vi "Scan action.vi"(8 "error in (no error)":errorcluster, 11 "SweepControl in":refnum<class "SMO.SweepControl.lvclass">) -> (0 "error out":errorcluster, 1 "Stop?":bool, 3 "SweepControl out":refnum<class "SMO.SweepControl.lvclass">)   [LabVIEW 2019, in "SMO.SweepControl.lvclass"]
uses:
  SMO.SweepControl.lvclass
  <userlib>/LevyLab/Lockin-Multichannel/Instrument.Lockin/Instrument.Lockin.lvclass
  Control Experiment/Control Experiment.lvclass
  <userlib>/LevyLab/Instrument Framework/Instrument Types/Cryostat/Typedefs/Magnet Mode--Enum.ctl
  <userlib>/LevyLab/Instrument Framework/Instrument Types/Cryostat/Instrument.Cryostat.lvclass
  <userlib>/LevyLab/Instrument Framework/Instrument Types/Strain/Instrument.Strain.lvclass
  <userlib>/LevyLab/Instrument Framework/Instrument Types/Delay Line/Instrument.DelayLine.lvclass
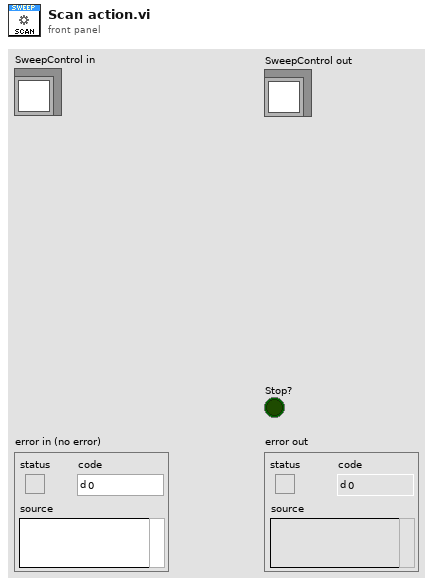
[diagram p1: front panel]
types:
  T1 = typedef "SMO.SweepControl.lvclass/Cluster - Sweep Control.ctl" = cluster{"Start":dbl, "End":dbl, "Step":dbl, "Rate":dbl, "wait (ms/mK)":u32, "Address":string, "Priority":T2, "Scan name":T3, "Post Actions":T4[], "channel":i32}
  T2 = typedef "SMO.SweepControl.lvclass/Enum - Priority.ctl" = enum16{"Priority 0", "Priority 1", "Priority 2", "Priority 3", "Priority 4", "Priority 5"}
  T3 = typedef "SMO.SweepControl.lvclass/Enum - Action.ctl" = enum16{"OFF", "time", "Lockin Amplitude", "Lockin Frequency", "Lockin Bias", "Delay", "Strain", "DAQ Bias", "Magnet Field", "Temperature", "MW f1", "MW f2", "MW Amplitude1", "MW Amplitude2"}
  T4 = typedef "SMO.SweepControl.lvclass/Enum - PostAction - 2.ctl" = enum16{"Do Nothing", "Wait (time)", "Wait (Temperature)", "Wait (<T ; B sweep)", "Wait (Magnet)"}
  T5 = typedef "SMO.SweepControl.lvclass/ScanParamters.ctl" = T6[]
  T6 = typedef "SMO.SweepControl.lvclass/Cluster - ScanParamters.ctl" = cluster{"Start":dbl, "End":dbl, "Step":dbl, "Rate":dbl, "Waveform type":enum16{"linear", "triangle", "power"}, "wait (ms or K)":dbl, "Address":string, "channel":i32}
  T7 = typedef "SMO.SweepControl.lvclass/ScanControl.ctl" = T8[]
  T8 = typedef "SMO.SweepControl.lvclass/Cluster - ScanControl.ctl" = cluster{"Priority":T2, "Scan name":T3}
  T9 = typedef "Control Experiment.lvclass/Instruments--cluster.ctl" = cluster{"KH7008":refnum<class "Instrument.KH7008.lvclass">[], "Lockin":refnum<class "Instrument.Lockin.lvclass">, "Temperature":refnum<class "Instrument.Cryostat.lvclass">, "Magnet":refnum<class "Instrument.Cryostat.lvclass">, "Rotator":refnum<class "Instrument.Cryostat.lvclass">, "Level":refnum<class "Instrument.Cryostat.lvclass">, "Capacitance Bridge":refnum<class "Instrument.CBridge.lvclass">, "Delay Line":refnum<class "Instrument.DelayLine.lvclass">, "Strain Cell":refnum<class "Instrument.Strain.lvclass">, "VNA":refnum<class "Instrument.VNA.lvclass">, "Voltage Source":refnum<class "Instrument.VSource.lvclass">}
  T10 = typedef "Instrument.Cryostat.lvclass/Magnet Mode--Enum.ctl" = enum16{"Persistent", "Driven"}
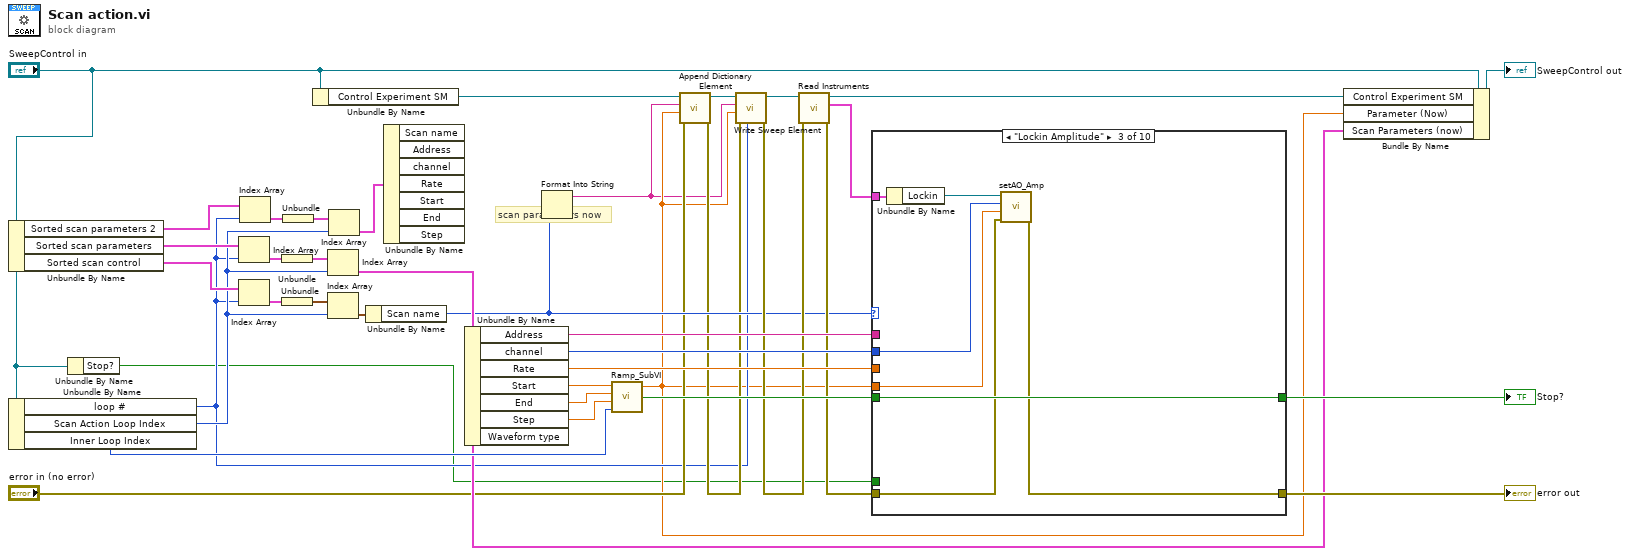
[diagram p0: block diagram]
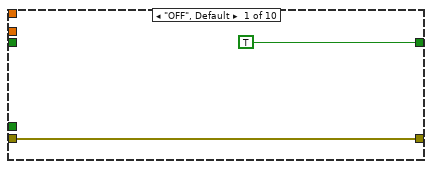
[diagram p2: hidden frame]
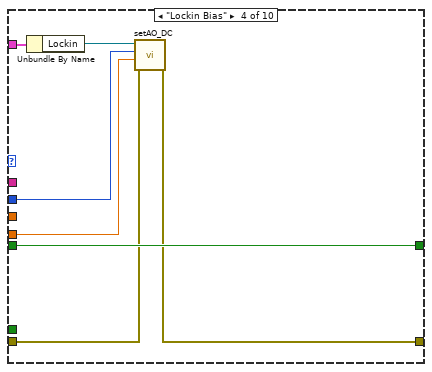
[diagram p4: hidden frame]
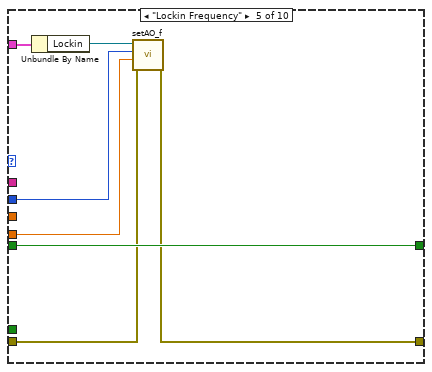
[diagram p5: hidden frame]
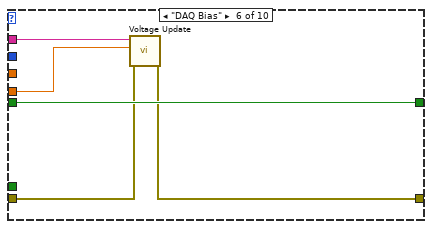
[diagram p6: hidden frame]
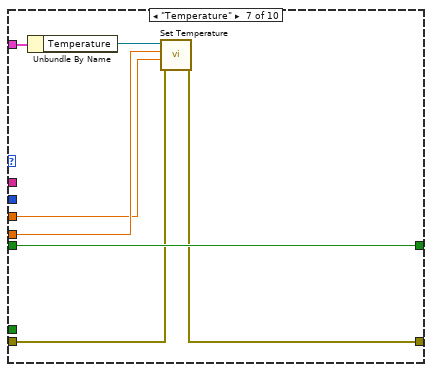
[diagram p7: hidden frame]
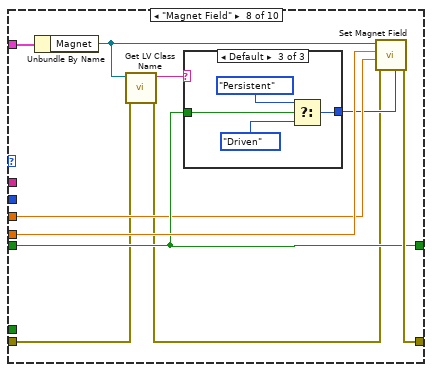
[diagram p8: hidden frame]
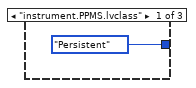
[diagram p9: hidden frame]
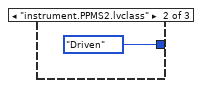
[diagram p10: hidden frame]
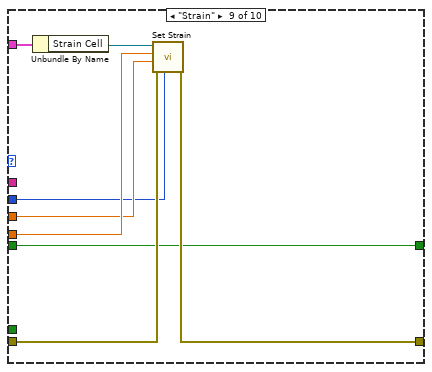
[diagram p11: hidden frame]
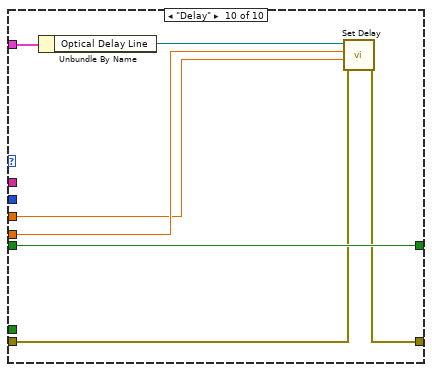
[diagram p12: hidden frame]
diagram:
  # "scan parameters now"
  n1 = Unbundle By Name("SweepControl in") -> ("Sorted scan parameters 2"=w13:cluster{"Scan parameters 2":T1[]}[], "Sorted scan parameters"=w30:cluster{T5}[], "Sorted scan control"=w24:cluster{T7}[])
  n2 = Unbundle By Name("SweepControl in") -> ("loop #"=w6:i32, "Scan Action Loop Index"=w14:i32, "Inner Loop Index"=w31:i32)
  n3 = Unbundle By Name("SweepControl in") -> ("Stop?"=w1:bool)
  n4 = Index Array(array=w30, index=w6) -> (element=w29:cluster{T5})
  n5 = Index Array(array=w24, index=w6) -> (element=w26:cluster{T7})
  n6 = Index Array(array=w13, index=w6) -> (element=w15:cluster{"Scan parameters 2":T1[]})
  n7 = Unbundle(w29) -> (w28:T5)
  n8 = Unbundle(w26) -> (w27:T7)
  n9 = Unbundle(w15) -> ("Scan parameters 2"=w16:T1[])
  n10 = Unbundle By Name("SweepControl in") -> ("Control Experiment SM"=w9:refnum<class "Control Experiment SM.lvclass">)
  n11 = Index Array(array=w28, index=w14) -> (element=w11:T6)
  n12 = Index Array(array=w27, index=w14) -> (element=w25:T8)
  n13 = Index Array(array=w16, index=w14) -> (element=w12:T1)
  n14 = Unbundle By Name(w25) -> ("Scan name"=w10:T3)
  n15 = Unbundle By Name(w12) -> ()  [unwired: 7 out]
  n16 = Unbundle By Name(w11) -> ("Address"=w37:string, "channel"=w39:i32, "Rate"=w34:dbl, "Start"=w36:dbl, "End"=w23:dbl, "Step"=w22:dbl)  [unwired: 1 out]
  n17 = Format Into String(w10) -> (resulting string=w3:string)  [unwired: 3 in, 1 out]
  n18 = call <userlib>:"Ramp_SubVI.vi"("index"=w31, "step"=w22, "end"=w23, "start"=w36) -> ("Stop?"=w35:bool, "Numeric"=w4:dbl)  [unwired: 1 in]
  n19 = call "Append Dictionary Element.vi"("error in (no error)"="error in (no error)", "value"=w4, "key"=w3, "Control Experiment in"=w9) -> ("error out"=w7:errorcluster, "Control Experiment out"=w5:refnum<class "Control Experiment.lvclass">)  [unwired: 6 in]
  n20 = call "Write Sweep Element.vi"("loop index"=w6, "error in (no error)"=w7, "value"=w4, "key"=w3, "Control Experiment in"=w5) -> ("error out"=w20:errorcluster, "Control Experiment out"=w21:refnum<class "Control Experiment.lvclass">)  [unwired: 5 in]
  n21 = call "Read Instruments.vi"("error in (no error)"=w20, "Control Experiment in"=w21) -> ("error out"=w19:errorcluster, "Instruments"=w17:T9, "Control Experiment out"=w18:refnum<class "Control Experiment.lvclass">)  [unwired: 7 in]
  n22 = case shown="\"Lockin Amplitude\"" w10 {
    tunnel: w39 -> [_ _ w47 w57 w64 _ _ _ w94 _]
    tunnel: [TRUE ("Stop?") w43 w50 w55 w62 w69 w76 w83 w93 w106] -> w38
    tunnel: w37 -> [_ _ _ _ _ w65 _ _ _ _]
    tunnel: w4 -> [_ _ w45 w56 w63 w68 w75 w85 w98 w102]
    tunnel: w35 -> [_ _ w50 w55 w62 w69 w76 w83 w93 w106]
    tunnel: w34 -> [_ _ _ _ _ _ w70 w82 w97 w101]
    tunnel: [w40 w42 w44 w54 w61 w67 w74 w86 w95 w103] -> w33
    tunnel: w17 -> [_ _ w46 w53 w58 _ w71 w84 w100 w107]
    tunnel: w19 -> [w40 w42 w49 w51 w59 w66 w72 w78 w96 w104]
    tunnel: w1 -> [_ w43 _ _ _ _ _ _ _ _]
    frame "OFF", Default {
    }
    frame "time" {
    }
    frame "Lockin Amplitude" {
      n23 = Unbundle By Name(w46) -> ("Lockin"=w48:refnum<class "Instrument.Lockin.lvclass">)
      n24 = call <userlib>:"setAO_Amp.vi"("error in (no error)"=w49, "Amplitude (V)"=w45, "AO Channel"=w47, "Instrument.Lockin in"=w48) -> ("error out"=w44:errorcluster)  [unwired: 6 in, 1 out]
    }
    frame "Lockin Bias" {
      n25 = Unbundle By Name(w53) -> ("Lockin"=w52:refnum<class "Instrument.Lockin.lvclass">)
      n26 = call <userlib>:"setAO_DC.vi"("error in (no error)"=w51, "DC (V)"=w56, "AO Channel"=w57, "Instrument.Lockin in"=w52) -> ("error out"=w54:errorcluster)  [unwired: 6 in, 1 out]
    }
    frame "Lockin Frequency" {
      n27 = Unbundle By Name(w58) -> ("Lockin"=w60:refnum<class "Instrument.Lockin.lvclass">)
      n28 = call <userlib>:"setAO_f.vi"("error in (no error)"=w59, "Frequency (Hz)"=w63, "AO Channel"=w64, "Instrument.Lockin in"=w60) -> ("error out"=w61:errorcluster)  [unwired: 6 in, 1 out]
    }
    frame "DAQ Bias" {
      n29 = call <userlib>:"Voltage Update.vi"("error in (no error)"=w66, "Voltage Output"=w68, "Physical Channel"=w65) -> ("error out"=w67:errorcluster)  [unwired: 6 in, 2 out]
    }
    frame "Temperature" {
      n30 = Unbundle By Name(w71) -> ("Temperature"=w73:refnum<class "Instrument.Cryostat.lvclass">)
      n31 = call-dynamic "Set Temperature.vi"("error in (no error)"=w72, "Rate (K/min)"=w70, "Temperature (K)"=w75, "Instrument.Cryostat in"=w73) -> ("error out"=w74:errorcluster)  [unwired: 6 in, 1 out]
    }
    frame "Magnet Field" {
      n32 = Unbundle By Name(w84) -> ("Magnet"=w80:refnum<class "Instrument.Cryostat.lvclass">)
      n33 = call <vilib>:"Get LV Class Name.vi"("error in (no error)"=w78, "object"=w80) -> ("error out"=w77:errorcluster, "class name"=w79:string)  [unwired: 8 in]
      n34 = case shown="Default" w79 {
        tunnel: w83 -> [_ _ w89]
        tunnel: [Magnet_Mode--Enum."Persistent" ("Mode") Magnet_Mode--Enum."Driven" ("Mode") w92] -> w81
        frame "instrument.PPMS.lvclass" {
        }
        frame "instrument.PPMS2.lvclass" {
        }
        frame Default {
          n35 = Select(t=Magnet_Mode--Enum."Persistent" ("Mode"), s=w89, f=Magnet_Mode--Enum."Driven" ("Mode")) -> (s? t:f=w92:T10)
        }
      }
      n36 = call-dynamic "Set Magnet Field.vi"("Mode"=w81, "error in (no error)"=w77, "Target Rate (T/min)"=w82, "Target Field (T)"=w85, "Instrument.Cryostat in"=w80) -> ("error out"=w86:errorcluster)  [unwired: 5 in, 1 out]
    }
    frame "Strain" {
      n37 = Unbundle By Name(w100) -> ("Strain Cell"=w99:refnum<class "Instrument.Strain.lvclass">)
      n38 = call-dynamic "Set Strain.vi"("Channel"=w94, "error in (no error)"=w96, "Slew (V/s)"=w97, "Strain (V)"=w98, "Instrument.Strain in"=w99) -> ("error out"=w95:errorcluster)  [unwired: 5 in, 1 out]
    }
    frame "Delay" {
      n39 = Unbundle By Name(w107) -> ("Optical Delay Line"=w105:refnum<class "Instrument.DelayLine.lvclass">)
      n40 = call-dynamic "Set Delay.vi"("error in (no error)"=w104, "Rate (ps/s)"=w101, "Delay (ps)"=w102, "Instrument.Delay in"=w105) -> ("error out"=w103:errorcluster)  [unwired: 6 in, 1 out]
    }
  }
  "Stop?" <- w38
  "error out" <- w33
  n41 = Bundle By Name(cluster="SweepControl in", "Control Experiment SM"=w18, "Parameter (Now)"=w4, "Scan Parameters (now)"=w11) -> (→"SweepControl out":refnum<class "SMO.SweepControl.lvclass">)
